vi "Separation des donnees.vi"() -> ()   [LabVIEW 2018]
panel:
  out "Numérique 2":i32
  out "Numérique":dbl
  in  "stop":bool
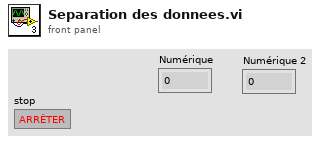
[diagram p1: front panel]
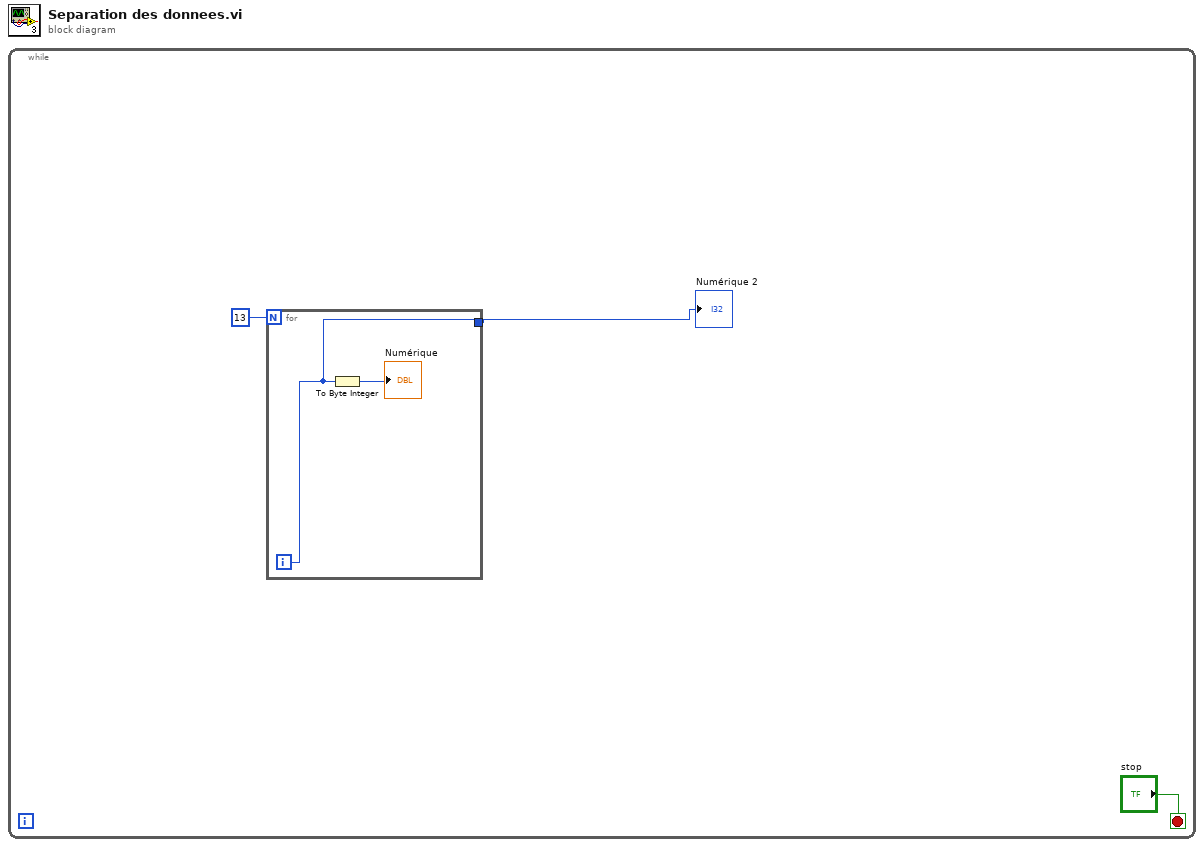
[diagram p0: block diagram]
diagram:
  n1 = while {
    stop <- "stop" stop-if-true
    n2 = for {
      N: 13 -> [_]
      tunnel: [w4] -> w1
      i -> [w4]
      n3 = To Byte Integer(number=w4) -> (8bit integer=→"Numérique":i8)
    }
    "Numérique 2" <- w1
  }
